vi "Init.vi"() -> (3 "No Op Msg out":refnum<class "No Op Msg.lvclass">)   [LabVIEW 2020, in "jettl.lvlib" / "No Op Msg.lvlib" / "No Op Msg.lvclass"]
uses:
  No Op Msg.lvclass
  Sender/Sender/Sender.lvclass
  No Op Msg.lvclass/No Op Msg.ctl
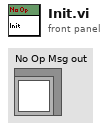
[diagram p1: front panel]
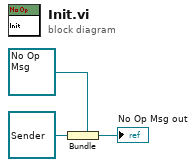
[diagram p0: block diagram]
diagram:
  n1 = Bundle "Bundle"(cluster=refnum<class "No Op Msg.lvclass"> refnum ("No Op Msg out"), refnum<class "Sender.lvclass"> refnum ("Sender")) -> (→"No Op Msg out":refnum<class "No Op Msg.lvclass">)
